vi "PXI-Enumerate Terminals.vi"(0 "ActiveDev":tag, 7 "String":string="(PFI[\\d]+)", 11 "error in (no error)":errorcluster) -> (4 "Full":string[](array[string]), 8 "Terminals":string[](array[string]), 15 "error out":errorcluster)   [LabVIEW 2020]
uses:
  <vilib>/regexp/Match Regular Expression.xnode
  <resource>/objmgr/daqmx.rc
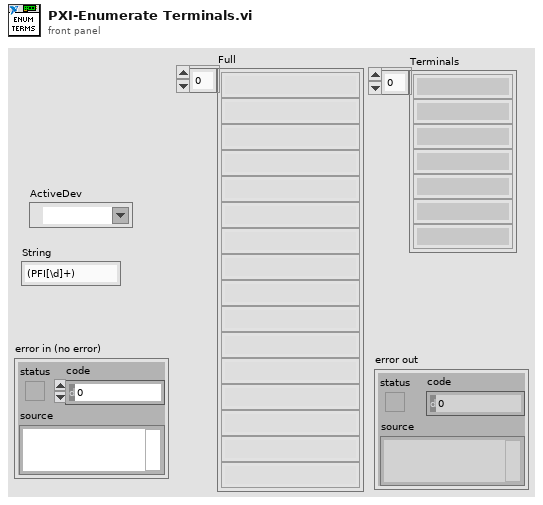
[diagram p1: front panel]
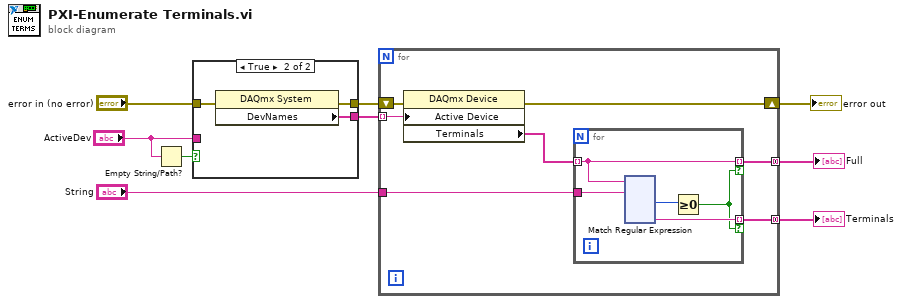
[diagram p0: block diagram]
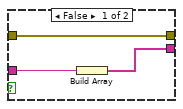
[diagram p2: hidden frame]
diagram:
  n1 = Empty String/Path?(string/path="ActiveDev") -> (empty?=w4:bool)
  n2 = case shown="True" w4 {
    tunnel: "ActiveDev" -> [w11 _]
    tunnel: "error in (no error)" -> [w12 w15]
    tunnel: [w12 w14] -> w2
    tunnel: [w10 w13] -> w1
    frame False {
      n3 = Build Array(w11) -> (w10:tag[])
    }
    frame True {
      n4 = property class="DAQmx System"(error in=w15) -> (error out=w14:errorcluster, "DevNames"=w13:tag[])  [unwired: 1 in, 1 out]
    }
  }
  n5 = for {
    tunnel: w1 -> [w21] mode=indexing
    tunnel: "String" -> [w18]
    tunnel: [w17] -> w8 mode=concatenating
    tunnel: [w16] -> w7 mode=concatenating
    shift-right: [w20] -> w9
    shift-left: w2 -> [w22]
    n6 = property class="DAQmx Device"(error in=w22, "Active Device"=w21) -> (error out=w20:errorcluster, "Terminals"=w19:tag[])  [unwired: 1 in, 1 out]
    n7 = for {
      tunnel: w19 -> [w27] mode=indexing
      tunnel: [w27] -> w17 mode=indexing if=w23
      tunnel: w18 -> [w26]
      tunnel: [w24] -> w16 mode=indexing if=w23
      n8 = xnode "Match Regular Expression"("input string"=w27, "regular expression"=w26) -> ("offset past match"=w25:i32, "submatch 1"=w24:string)  [unwired: 4 in, 4 out]
      n9 = Greater Or Equal To 0?(x=w25) -> (x >= 0?=w23:bool)
    }
  }
  "error out" <- w9
  "Full" <- w8
  "Terminals" <- w7
